vi "ObjectsFGV.vi"(10 "read?":bool, 11 "Classes":T1) -> (3 "output cluster":T1)   [LabVIEW 2017]
uses:
  Drive/Classes.ctl
  Drive/Drive.lvclass
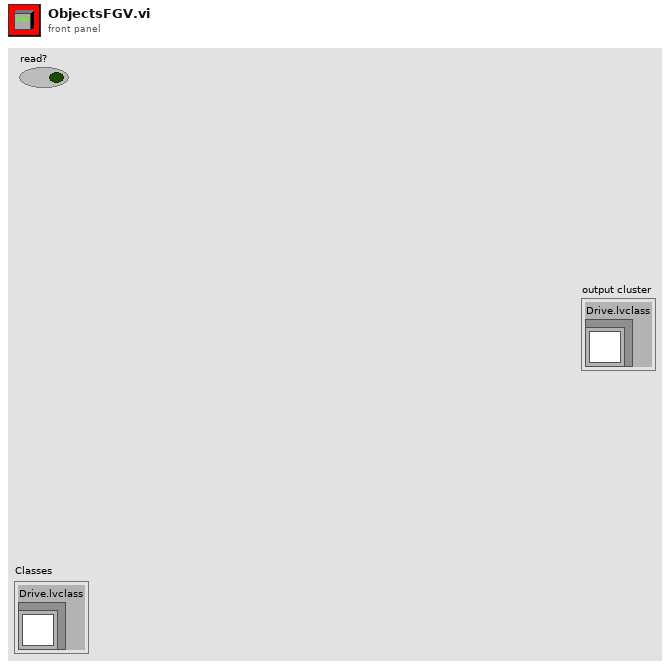
[diagram p1: front panel]
types:
  T1 = typedef "Classes.ctl" = cluster{"Drive.lvclass":refnum<class "Drive.lvclass">}
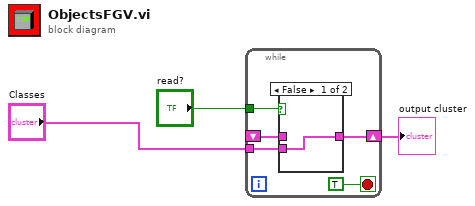
[diagram p0: block diagram]
diagram:
  n1 = while {
    shift-right: [w6] -> w3
    shift-left: _ -> [w8]
    tunnel: "Classes" -> [w7]
    tunnel: "read?" -> [w4]
    stop <- TRUE stop-if-true
    n2 = case shown="False" w4 {
      tunnel: w8 -> [_ w10]
      tunnel: [w9 w10] -> w6
      tunnel: w7 -> [w9 _]
      frame False {
      }
      frame True {
      }
    }
  }
  "output cluster" <- w3
